vi "licor_test.vi"() -> ()   [LabVIEW 2011]
uses:
  <vilib>/addons/database/Connection.llb/DB Tools Open Connec (String).vi
  <vilib>/addons/database/Auxilliary.llb/DB Tools Format Datetime String (Time Stamp).vi
  <vilib>/addons/database/NI_Database_API.lvlib
  Program Files (x86)/National Instruments/LabVIEW 2011/resource/objmgr/daqmx.rc
panel:
  out "Cluster":variant
  out "output array":refnum<k21>[](array[refnum])
  out "Channels":refnum<k21>[](array[refnum])
  out "decimal integer string":string
  out "Array":dbl[](array[numeric])
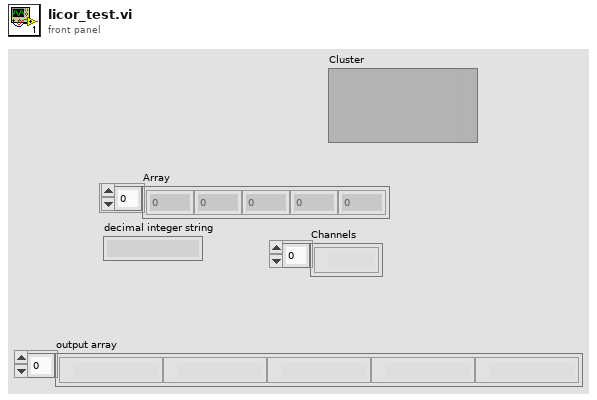
[diagram p1: front panel]
types:
  T1 = typedef "NI_Database_API.lvlib/Conn ObjectReference.ctl" = refnum<k1>
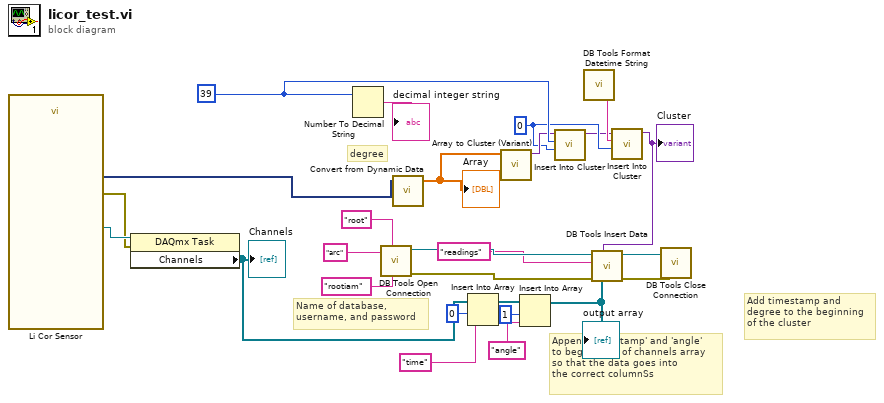
[diagram p0: block diagram]
diagram:
  w4 = 0
  w6 = 39
  # "Append 'timestamp' and 'angle'\nto beginnging of channels array\nso that the data goes into\nthe correct columnSs"
  # "degree"
  # "Name of database,\nusername, and password"
  # "Add timestamp and \ndegree to the beginning\nof the cluster"
  n1 = call "Li Cor Sensor"() -> ("task out"=w16:refnum<k21>, "data"=w26:dynamicdata, "error out"=w15:errorcluster)  [unwired: 16 in, 1 out]
  n2 = property class="DAQmx Task"(reference=w16, error in=w15) -> ("Channels"=w8:refnum<k21>[])  [unwired: 2 out]
  "Channels" <- w8
  n3 = Number To Decimal String(number=w6) -> (decimal integer string=→"decimal integer string":string)  [unwired: 1 in]
  n4 = call-poly <vilib>:"DB Tools Open Connection.vi"("password"="rootiam", "userID"="root", "connection information"="arc") -> ("error out"=w23:errorcluster, "connection reference"=w24:T1)  [unwired: 5 in]
  n5 = call "Convert from Dynamic Data"("Dynamic Data Type"=w26) -> ("Array"=w7:dbl[])  [unwired: 3 in]
  "Array" <- w7
  n6 = Insert Into Array(array=w8, index=0, new element="time") -> (w12:refnum<k21>[])
  n7 = call <vilib>:"Array to Cluster (Variant).vi"("Array"=w7) -> ("Cluster"=w5:variant)  [unwired: 9 in, 1 out]
  n8 = Insert Into Array(array=w12, index=1, new element="angle") -> (w9:refnum<k21>[])
  "output array" <- w9
  n9 = call <vilib>:"Insert Into Cluster.vi"("Index"=w4, "Element"=w6, "Cluster"=w5) -> ("Cluster w/ Element Inserted"=w2:variant)  [unwired: 5 in, 3 out]
  n10 = call-poly <vilib>:"DB Tools Format Datetime String.vi"() -> ("date/time string"=w3:string)  [unwired: 1 in]
  n11 = call <vilib>:"Insert Into Cluster.vi"("Index"=w4, "Element"=w3, "Cluster"=w2) -> ("Cluster w/ Element Inserted"=w1:variant)  [unwired: 5 in, 3 out]
  "Cluster" <- w1
  n12 = call <vilib>:"DB Tools Insert Data.vi"("data"=w1, "error in (no error)"=w23, "columns"=w9, "table"="readings", "connection reference"=w24) -> ("error out"=w20:errorcluster, "connection reference out"=w21:T1)  [unwired: 5 in]
  n13 = call <vilib>:"DB Tools Close Connection.vi"("error in (no error)"=w20, "connection reference"=w21) -> ()  [unwired: 5 in, 1 out]
